vi "Calculator.vi"() -> ()   [LabVIEW 2021]
uses:
  Operator.ctl
  <vilib>/gmath/NI_Gmath.lvlib
  a4a78011-f8a5-4b46-8114-8a867b825412.vi
  Digits.ctl
  Operators.ctl
panel:
  in  "Stop":bool
  out "Display":string
  in  "Operators":T1
  in  "Digits":T2
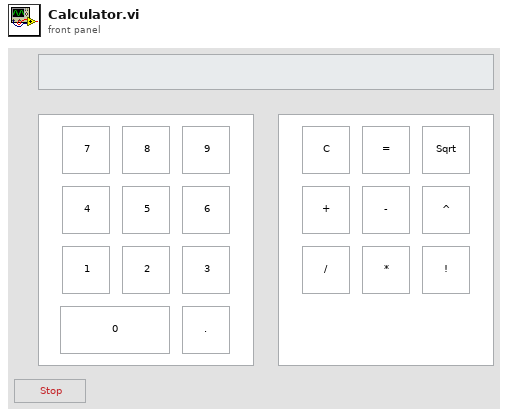
[diagram p1: front panel]
types:
  T1 = typedef "Operators.ctl" = cluster{"clear":bool, "equal":bool, "sqrt":bool, "add":bool, "sub":bool, "pwr":bool, "div":bool, "mul":bool, "fact":bool}
  T2 = typedef "Digits.ctl" = cluster{"Button 0":bool, "Button 1":bool, "Button 2":bool, "Button 3":bool, "Button 4":bool, "Button 5":bool, "Button 6":bool, "Button 7":bool, "Button 8":bool, "Button 9":bool, "Button 10":bool}
  T3 = typedef "Operator.ctl" = enum16{"add", "sub", "mul", "div", "pwr", "sqrt", "fact", "equal", "clear"}
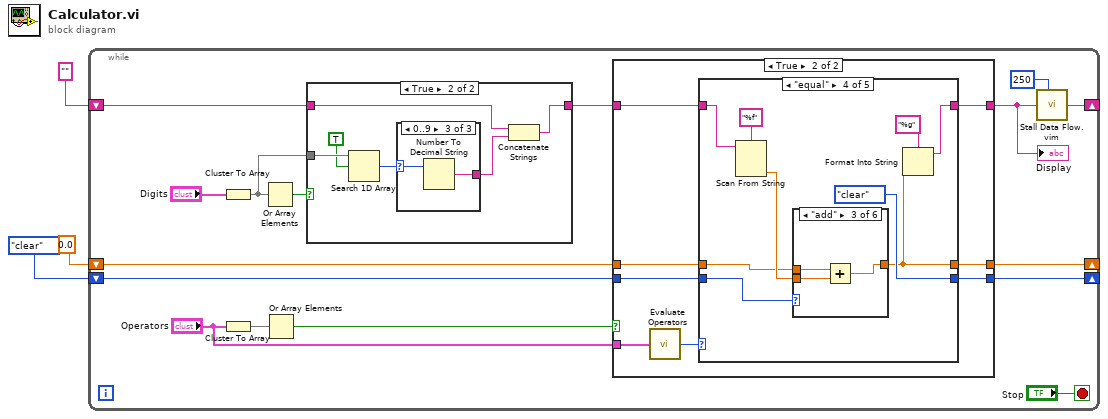
[diagram p0: block diagram]
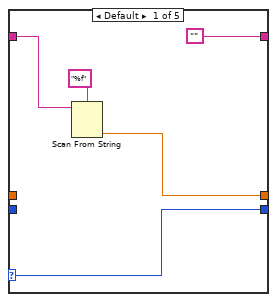
[diagram p3: hidden frame]
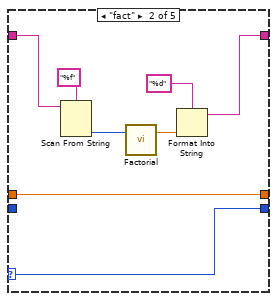
[diagram p4: hidden frame]
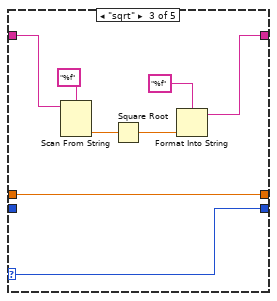
[diagram p5: hidden frame]
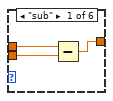
[diagram p6: hidden frame]
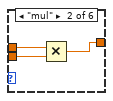
[diagram p7: hidden frame]
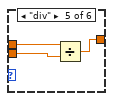
[diagram p9: hidden frame]
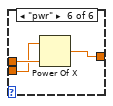
[diagram p10: hidden frame]
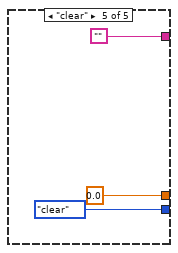
[diagram p11: hidden frame]
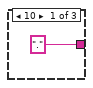
[diagram p13: hidden frame]
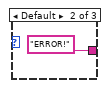
[diagram p14: hidden frame]
diagram:
  n1 = while {
    shift-right: [w6] -> _
    shift-left: "" -> [w15]
    shift-right: [w9] -> _
    shift-left: 0.0 -> [w8]
    shift-right: [w7] -> _
    shift-left: Operator."clear" ("Operator") -> [w4]
    stop <- "Stop" stop-if-true
    n2 = Cluster To Array(cluster="Digits") -> (array=w17:bool[])
    n3 = Cluster To Array(cluster="Operators") -> (array=w19:bool[])
    n4 = Or Array Elements(Boolean array=w17) -> (logical OR=w14:bool)
    n5 = Or Array Elements(Boolean array=w19) -> (logical OR=w12:bool)
    n6 = case shown="True" w14 {
      tunnel: w17 -> [_ w86]
      tunnel: [w80 w82] -> w13
      tunnel: w15 -> [w80 w83]
      frame False {
      }
      frame True {
        n7 = Search 1D Array(1D array=w86, element=TRUE) -> (index of element=w81:i32)  [unwired: 1 in]
        n8 = case shown="0..9" w81 {
          selector: w81 -> [_ _ w89]
          tunnel: ["." "ERROR!" w90] -> w84
          frame 10 {
          }
          frame Default {
          }
          frame 0..9 {
            n9 = Number To Decimal String(number=w89) -> (decimal integer string=w90:string)  [unwired: 1 in]
          }
        }
        n10 = Concatenate Strings(w83, w84) -> (w82:string)
      }
    }
    n11 = case shown="True" w12 {
      tunnel: w13 -> [w22 w30]
      tunnel: "Operators" -> [_ w28]
      tunnel: [w22 w25] -> w10
      tunnel: [w21 w29] -> w9
      tunnel: w8 -> [w21 w24]
      tunnel: [w20 w26] -> w7
      tunnel: w4 -> [w20 w23]
      frame False {
      }
      frame True {
        n12 = call "Evaluate Operators.vi"("Operators"=w28) -> ("Operator"=w27:T3)  [unwired: 14 in]
        n13 = case shown="\"equal\"" w27 {
          selector: w27 -> [w31 w41 w49 _ _]
          tunnel: w30 -> [w33 w42 w50 w59 _]
          tunnel: [w34 w39 w47 w54 0.0] -> w29
          tunnel: [w31 w41 w49 Operator."clear" ("Operator") Operator."clear" ("Operator")] -> w26
          tunnel: ["" w37 w45 w53 ""] -> w25
          tunnel: w24 -> [_ w39 w47 w56 _]
          tunnel: w23 -> [_ _ _ w52 _]
          frame Default {
            n14 = Scan From String(format string="%f", input string=w33) -> (output 1=w34:dbl)  [unwired: 3 in, 3 out]
          }
          frame "fact" {
            n15 = Scan From String(format string="%f", input string=w42) -> (output 1=w40:i32)  [unwired: 3 in, 3 out]
            n16 = call <vilib>:"Factorial.vi"("n"=w40) -> ("n!"=w38:dbl)  [unwired: 2 in]
            n17 = Format Into String(format string="%d", w38) -> (resulting string=w37:string)  [unwired: 2 in, 1 out]
          }
          frame "sqrt" {
            n18 = Scan From String(format string="%f", input string=w50) -> (output 1=w48:dbl)  [unwired: 3 in, 3 out]
            n19 = Square Root(x=w48) -> (sqrt(x)=w46:dbl)
            n20 = Format Into String(format string="%f", w46) -> (resulting string=w45:string)  [unwired: 2 in, 1 out]
          }
          frame "equal" {
            n21 = Scan From String(format string="%f", input string=w59) -> (output 1=w57:dbl)  [unwired: 3 in, 3 out]
            n22 = case shown="\"add\"" w52 {
              tunnel: w57 -> [w63 w65 w68 _ w72 w75]
              tunnel: w56 -> [w62 w66 w69 w70 w73 w76]
              tunnel: [w61 w64 w67 w70 w71 w74] -> w54
              frame "sub" {
                n23 = Subtract(x=w62, y=w63) -> (x-y=w61:dbl)
              }
              frame "mul" {
                n24 = Multiply(x=w66, y=w65) -> (x*y=w64:dbl)
              }
              frame "add" {
                n25 = Add(x=w69, y=w68) -> (x+y=w67:dbl)
              }
              frame Default {
              }
              frame "div" {
                n26 = Divide(x=w73, y=w72) -> (x/y=w71:dbl)
              }
              frame "pwr" {
                n27 = Power Of X(1:w76, 2:w75) -> (0:w74:dbl)
              }
            }
            n28 = Format Into String(format string="%g", w54) -> (resulting string=w53:string)  [unwired: 2 in, 1 out]
          }
          frame "clear" {
          }
        }
      }
    }
    "Display" <- w10
    n29 = call "Stall Data Flow.vim"("value in"=w10, "milliseconds to wait"=u32 250) -> ("value out"=w6:string)  [unwired: 1 out]
  }
